vi "Chirp Train (G3)-Initialize.vi"(0 "Chirp Train in":T3, 5 "Level":T1, 7 "Sampling rate (Hz)":dbl, 9 "Npts":i32, 11 "error in (no error)":errorcluster) -> (4 "Chirp Train out":T3, 15 "error out":errorcluster)   [LabVIEW 2020]
uses:
  Waveform VIs/Chirp Train VIs/Chirp Train.ctl
  Waveform VIs/Chirp Train VIs/Chirp Train Params.ctl
  XControls/Level (G3)/Level Data.ctl
  XControls/Level (G3)/Level Units (G3).ctl
  XControls/Level (G3)/Level (G3).xctl
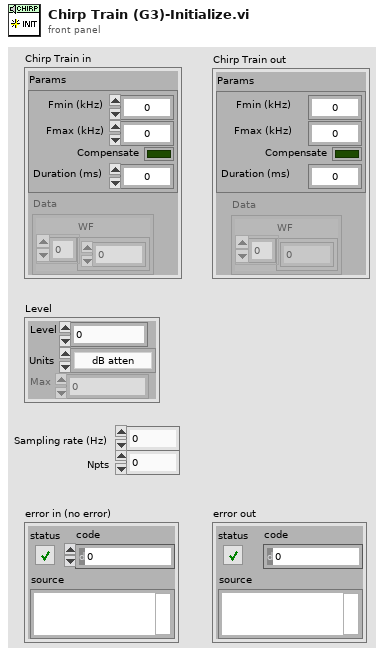
[diagram p1: front panel]
types:
  T1 = typedef "Level (G3).xctl/Level Data.ctl" = cluster{"Level":dbl, "Units":T2, "Max":dbl, "Data":cluster{"Multiplier":dbl, "Cal File":path, "Cal":cluster{"Freq (Hz)":dbl[], "Mag (dB SPL)":dbl[], "Phase (deg)":dbl[]}, "audiogram":path}}
  T2 = typedef "Level (G3).xctl/Level Units (G3).ctl" = enum16{"dB atten", "dB SPL", "dB re 1 Vrms", "dB V/Hz½", "mW", "dB HL", "Volts", "dB mW"}
  T3 = typedef "Chirp Train.ctl" = cluster{"Params":T4, "Data":cluster{"WF":dbl[]}}
  T4 = typedef "Chirp Train Params.ctl" = cluster{"Fmin (kHz)":dbl, "Fmax (kHz)":dbl, "Compensate":bool, "Duration (ms)":dbl}
  T5 = cluster{"Freq (Hz)":dbl[], "Mag (dB SPL)":dbl[], "Phase (deg)":dbl[]}
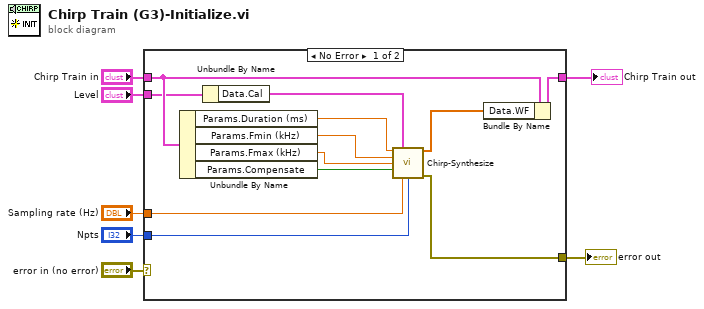
[diagram p0: block diagram]
diagram:
  n1 = case shown="No Error" "error in (no error)" {
    selector: "error in (no error)" -> [_ w20]
    tunnel: [w9 w20] -> w3
    tunnel: "Chirp Train in" -> [w19 _]
    tunnel: [w18 _] -> w5
    tunnel: "Sampling rate (Hz)" -> [w11 _]
    tunnel: "Npts" -> [w10 _]
    tunnel: "Level" -> [w17 _]
    frame No Error {
      n2 = Unbundle By Name(w19) -> ("Params.Duration (ms)"=w15:dbl, "Params.Fmin (kHz)"=w14:dbl, "Params.Fmax (kHz)"=w13:dbl, "Params.Compensate"=w12:bool)
      n3 = Unbundle By Name(w17) -> ("Data.Cal"=w16:T5)
      n4 = call "Chirp-Synthesize.vi"("Duration (ms)"=w15, "Cal"=w16, "Fmin (kHz)"=w14, "Fmax (kHz)"=w13, "Compensate"=w12, "Sampling rate (Hz)"=w11, "Npts"=w10) -> ("Data.WF"=w8:dbl[], "error out"=w9:errorcluster)  [unwired: 7 in]
      n5 = Bundle By Name(cluster=w19, "Data.WF"=w8) -> (w18:T3)
    }
    frame Error {
    }
  }
  "Chirp Train out" <- w5
  "error out" <- w3
